vi "authenticateClient.vi"(8 "error in (no error)":errorcluster, 10 "Computer Name":string, 11 "tcpServer in":refnum<class "TcpServer.lvclass">) -> (0 "error out":errorcluster, 2 "authenticate":bool, 3 "tcpServer out":refnum<class "TcpServer.lvclass">)   [LabVIEW 2018, in "TcpServer.lvclass"]
doc: "Authenticate Tcp Client, getting Client info from configServer.vi."
uses:
  TcpServer.lvclass
  TcpServer.lvclass/TcpServer.ctl
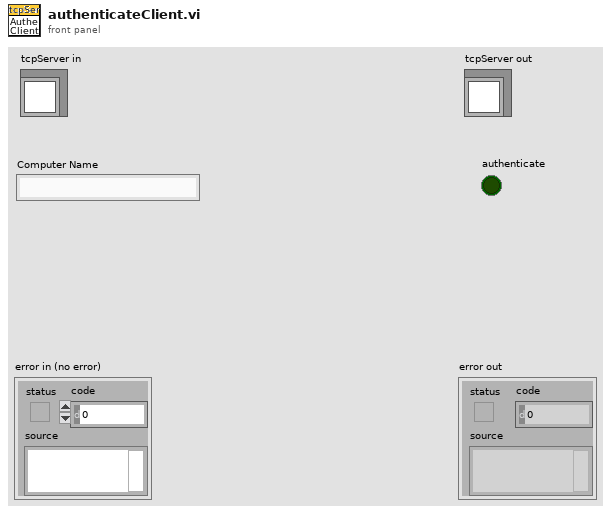
[diagram p1: front panel]
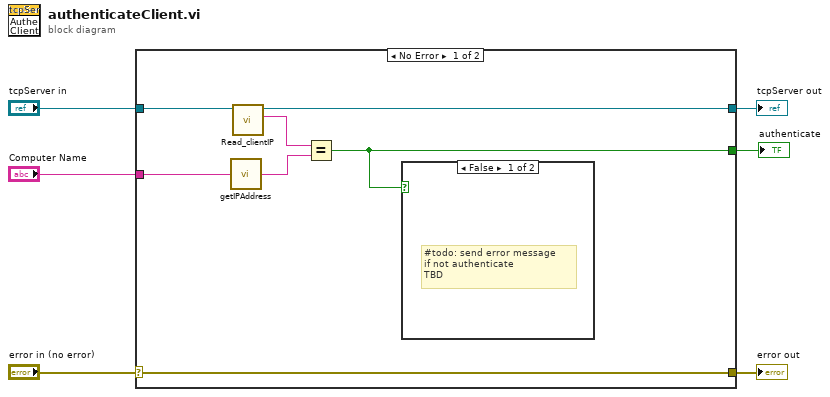
[diagram p0: block diagram]
diagram:
  n1 = case shown="No Error" "error in (no error)" {
    selector: "error in (no error)" -> [w13 w15]
    tunnel: [w13 w15] -> w5
    tunnel: [w11 w14] -> w3
    tunnel: "tcpServer in" -> [w12 w14]
    tunnel: [w7 _] -> w2
    tunnel: "Computer Name" -> [w10 _]
    frame No Error {
      n2 = call "getIPAddress.vi"("Computer Name"=w10) -> ("IP Address"=w8:string)
      n3 = call "Read_clientIP.vi"("tcpServer in"=w12) -> ("clientIP"=w9:string, "tcpServer out"=w11:refnum<class "TcpServer.lvclass">)  [unwired: 8 in, 1 out]
      n4 = Equal?(x=w9, y=w8) -> (x = y?=w7:bool)
      n5 = case shown="False" w7 {
        frame False {
          # "#todo: send error message\nif not authenticate\nTBD"
        }
        frame True {
          # "#todo: send ack to client\nTBD"
        }
      }
    }
    frame Error {
    }
  }
  "error out" <- w5
  "tcpServer out" <- w3
  "authenticate" <- w2
